vi "Run Client.vi"() -> ()   [LabVIEW 2020, in "Client.lvlib"]
uses:
  Client.lvlib
  Measurement Service Client V2/RPC Messages/ni_measurementlink_measurement_v2_MeasureRequest.ctl
  Measurement Service Client V2/RPC Messages/google_protobuf_Any.ctl
  Measurement Service Client V2/RPC Messages/ni_measurementlink_PinMapContext.ctl
  Service/Service/Measurement Results.ctl
  Service/Service/Measurement Configuration.ctl
  152ea591-9aaf-4835-9cf9-cce158645c57.vi
  045899de-a912-426a-8a5d-a949b9672173.vi
  <vilib>/gRPC/LabVIEW gRPC Library/Server API/Translate Protobuf Error.vi
  <vilib>/AdvancedString/1D String Array to Delimited String.vi
  <vilib>/gRPC/LabVIEW gRPC Library/Server API/Server/Get Server DLL Path.vi
  <vilib>/gRPC/LabVIEW gRPC Library/grpc-lvsupport-release.lvlib
  Measurement Service Client V2/Measurement Service Client V2.lvlib
  Service/Service/Service.lvlib
panel:
  in  "time in seconds":dbl=5.0
  out "random numbers":dbl[](graph)
  out "elapsed time":dbl
  out "status":string
  in  "stop":bool
  out "error out":errorcluster
  in  "service to run":string="ServiceforLabVIEWClient_LabVIEW"
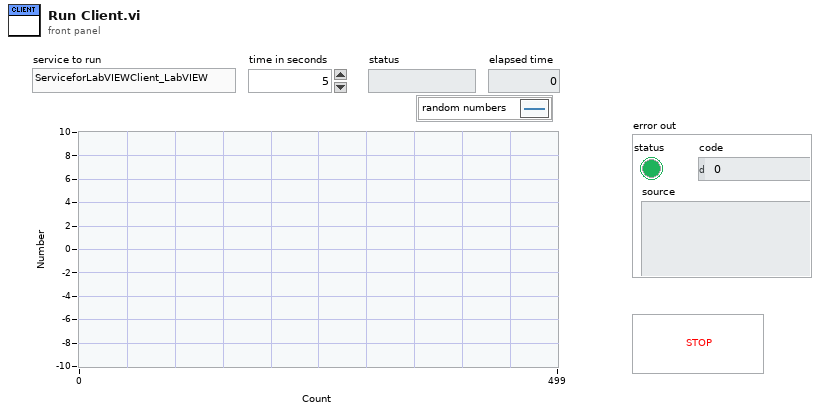
[diagram p1: front panel]
types:
  T1 = typedef "Service.lvlib/Measurement Configuration.ctl" = cluster{"time in seconds":dbl}
  T2 = typedef "Service.lvlib/Measurement Results.ctl" = cluster{"random numbers":dbl[], "status":string, "elapsed time":dbl}
  T3 = typedef "Measurement Service Client V2.lvlib/ni_measurementlink_measurement_v2_MeasureRequest.ctl" = cluster{"configuration_parameters":T4, "pin_map_context":T5}
  T4 = typedef "Measurement Service Client V2.lvlib/google_protobuf_Any.ctl" = cluster{"type_url":string, "value":u8[]}
  T5 = typedef "Measurement Service Client V2.lvlib/ni_measurementlink_PinMapContext.ctl" = cluster{"pin_map_id":string, "sites":i32[]}
  T6 = typedef "grpc-lvsupport-release.lvlib/grpcId.ctl" = u64
  T7 = typedef "grpc-lvsupport-release.lvlib/Message Metadata.ctl" = cluster{"Version":i32, "Name":string, "Type Url":string, "Elements":T8[], "Has Oneof":bool}
  T8 = typedef "grpc-lvsupport-release.lvlib/Message Element Metadata.ctl" = cluster{"Field Name":string, "Embedded Message Name":string, "Protobuf Index":i32, "MessageElementType":T9, "Repeated":bool, "Is in Oneof":bool, "Oneof Container Name":string}
  T9 = typedef "grpc-lvsupport-release.lvlib/Message Element Type.ctl" = enum32{"Int32Value", "FloatValue", "DoubleValue", "BoolValue", "StringValue", "MessageValue", "Int64Value", "UInt32Value", "UInt64Value", "EnumValue", "Bytes", "Fixed64", "Fixed32", "SFixed64", "SFixed32", "SInt64", "SInt32"}
  T10 = typedef "grpc-lvsupport-release.lvlib/Any.ctl" = cluster{"Type Url":string, "Bytes":u8[]}
  T11 = typedef "Measurement Service Client V2.lvlib/ni_measurementlink_measurement_v2_MeasureResponse.ctl" = cluster{"outputs":T4}
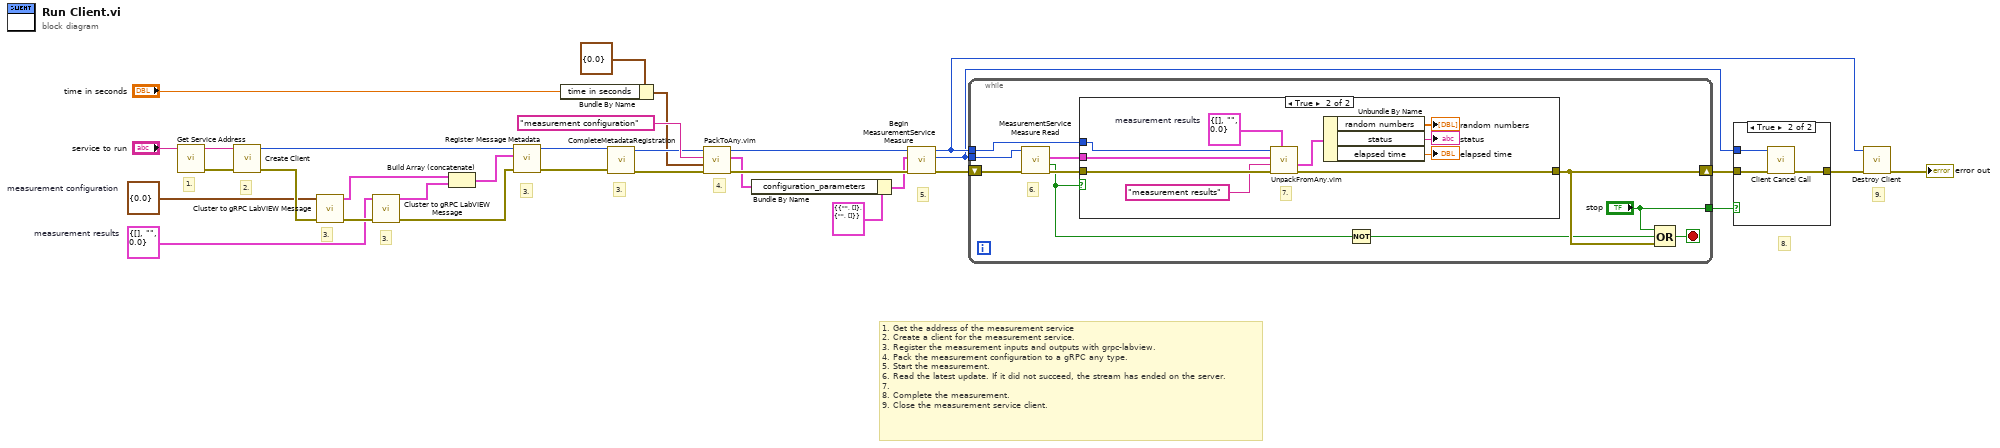
[diagram p0: block diagram]
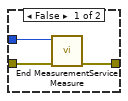
[diagram p2: hidden frame]
diagram:
  w8 = T1 {"time in seconds"=0.0}  # measurement configuration
  w9 = T2 {"random numbers"=[], "status"="", "elapsed time"=0.0}  # measurement results
  # "3."
  # "3."
  # "3."
  # "9."
  # "8."
  # "5."
  # "4."
  # "3."
  # "1. Get the address of the measurement service\n2. Create a client for the measurement service.\n3. Register the measurement inputs and outputs with grpc-labview.\n4. Pack the measurement configuration to a gRPC any type.\n5. Start the measurement.\n6. Read the latest update. If it did not succeed, the stream has ended on the server.\n7. \n8. Complete the measurement.\n9. Close the measurement service client."
  # "2."
  # "1."
  n1 = call "Get Service Address.vi"("service to run"="service to run") -> ("error out"=w29:errorcluster, "service address"=w14:string)  [unwired: 9 in]
  n2 = call "Create Client.vi"("error in"=w29, "address"=w14) -> ("error out"=w12:errorcluster, "gRPC ID Out"=w28:T6)  [unwired: 8 in]
  n3 = call <vilib>:"Cluster to gRPC LabVIEW Message.vi"("error in"=w12, "Cluster"=w8) -> ("error out"=w11:errorcluster, "gRPC Message Metadata []"=w32:T7[])  [unwired: 7 in, 1 out]
  n4 = call <vilib>:"Cluster to gRPC LabVIEW Message.vi"("error in"=w11, "Cluster"=w9) -> ("error out"=w10:errorcluster, "gRPC Message Metadata []"=w31:T7[])  [unwired: 7 in, 1 out]
  n5 = Build Array (concatenate)(w32, w31) -> (w30:T7[])
  n6 = call <vilib>:"Register Message Metadata.vi"("error in"=w10, "Messages"=w30, "gRPCid in"=w28) -> ("error out"=w25:errorcluster, "gRPCid out"=w26:T6)  [unwired: 7 in]
  n7 = Bundle By Name(cluster=T1 {"time in seconds"=0.0} ("Measurement Configuration"), "time in seconds"="time in seconds") -> (w5:T1)
  n8 = call <vilib>:"CompleteMetadataRegistration.vi"("error in"=w25, "gRPC ID in"=w26) -> ("error out"=w13:errorcluster, "gRPC ID Out"=w23:T6)  [unwired: 8 in]
  n9 = call "PackToAny.vim"("error in"=w13, "Data To Pack"=w5, "Message Type"="measurement configuration", "gRPCid in"=w23) -> ("error out"=w22:errorcluster, "Any"=w19:T10, "gRPCid out"=w21:u64)  [unwired: 5 in]
  n10 = Bundle By Name(cluster=T3 {"configuration_parameters"={"type_url"="", "value"=[]}, "pin_map_context"={"pin_map_id"="", "sites"=[]}} ("Request Data"), "configuration_parameters"=w19) -> (w16:T3)
  n11 = call "Begin MeasurementService Measure.vi"("error in"=w22, "Request Data"=w16, "gRPC ID"=w21) -> ("error out"=w18:errorcluster, "Call Id Out"=w4:T6, "gRPC ID out"=w17:T6)  [unwired: 6 in]
  n12 = while {
    tunnel: w4 -> [w39]
    tunnel: w17 -> [w38]
    shift-right: [w36] -> w2
    shift-left: w18 -> [w40]
    tunnel: ["stop"] -> w3
    stop <- w42 stop-if-true
    # "6."
    n13 = call "MeasurementService Measure Read.vi"("error in"=w40, "Call ID in"=w39) -> ("error out"=w37:errorcluster, "Success"=w35:bool, "Response Data"=w41:T11)  [unwired: 6 in, 1 out]
    n14 = case shown="True" w35 {
      tunnel: w41 -> [_ w52]
      tunnel: w38 -> [_ w51]
      tunnel: w37 -> [w43 w50]
      tunnel: [w43 w49] -> w36
      frame False {
      }
      frame True {
        w47 = T2 {"random numbers"=[], "status"="", "elapsed time"=0.0}  # measurement results
        # "7."
        n15 = call "UnpackFromAny.vim"("Data Type"=w47, "error in"=w50, "Message Type"="measurement results", "Any"=w52, "gRPCid in"=w51) -> ("error out"=w49:errorcluster, "Unpacked Value"=w53:T2)  [unwired: 4 in, 1 out]
        n16 = Unbundle By Name(w53) -> ("random numbers"=→"random numbers":dbl[], "status"=→"status":string, "elapsed time"=→"elapsed time":dbl)
      }
    }
    n17 = Not(x=w35) -> (.not. x?=w34:bool)
    n18 = Compound Arithmetic op=OR("stop", w34, w36) -> (w42:bool)
  }
  n19 = case shown="True" w3 {
    tunnel: w4 -> [w55 w59]
    tunnel: w2 -> [w56 w58]
    tunnel: [w54 w57] -> w1
    frame False {
      n20 = call "End MeasurementService Measure.vi"("error in"=w56, "Call ID in"=w55) -> ("error out"=w54:errorcluster)  [unwired: 8 in, 1 out]
    }
    frame True {
      n21 = call <vilib>:"Client Cancel Call.vi"("error in"=w58, "Call ID in"=w59) -> ("error out"=w57:errorcluster)  [unwired: 7 in, 2 out]
    }
  }
  n22 = call "Destroy Client.vi"("error in"=w1, "gRPC ID"=w17) -> ("error out"=→"error out":errorcluster)  [unwired: 9 in]
